vi "Read Analog In.vi"(8 "error in":errorcluster, 11 "PLC in":refnum<class "PLC.lvclass">) -> (0 "error out":errorcluster, 2 "Analog In":dbl[](array[numeric]), 3 "PLC out":refnum<class "PLC.lvclass">)   [LabVIEW 2018, in "PLC.lvlib" / "PLC.lvclass"]
uses:
  PLC.lvclass
  PLC.lvclass/PLC.ctl
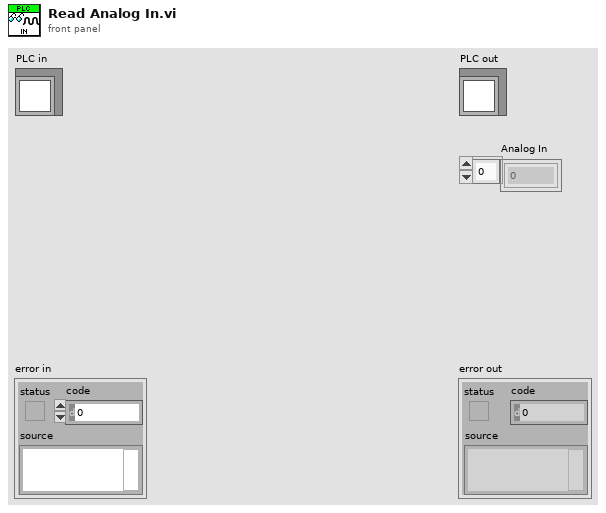
[diagram p1: front panel]
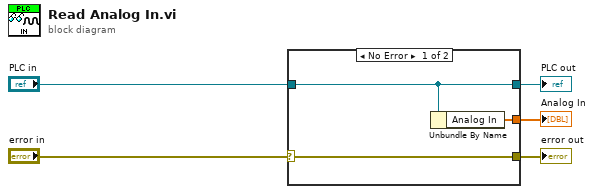
[diagram p0: block diagram]
diagram:
  n1 = case shown="No Error" "error in" {
    selector: "error in" -> [w8 w9]
    tunnel: [w8 w9] -> w5
    tunnel: [w7 w10] -> w4
    tunnel: "PLC in" -> [w7 w10]
    tunnel: [w6 _] -> w3
    frame No Error {
      n2 = Unbundle By Name(w7) -> ("Analog In"=w6:dbl[])
    }
    frame Error {
    }
  }
  "error out" <- w5
  "PLC out" <- w4
  "Analog In" <- w3
